vi "IN_1_BIT.vi"(11 "String":string) -> (0 "error out":errorcluster, 3 "data":bool)   [LabVIEW 2017]
uses:
  <vilib>/DAQmx/read.llb/DAQmx Read (Digital Bool 1Line 1Point).vi
  <vilib>/DAQmx/create/channels.llb/DAQmx Create Channel (DO-Digital Output).vi
  <vilib>/DAQmx/miscellaneous.llb/DAQmx Fill In Error Info.vi
panel:
  in  "lines":tag
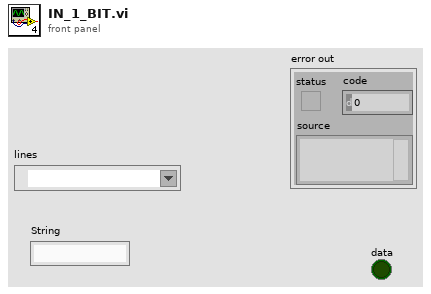
[diagram p1: front panel]
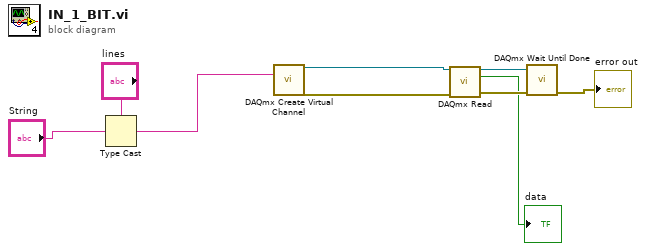
[diagram p0: block diagram]
diagram:
  n1 = Type Cast(type="lines", x="String") -> (*(type *) &x=w7:tag)
  n2 = call-poly <vilib>:"DAQmx Create Virtual Channel.vi"("lines"=w7) -> ("task out"=w5:refnum<k21>, "error out"=w4:errorcluster)  [unwired: 13 in]
  n3 = call-poly <vilib>:"DAQmx Read.vi"("task/channels in"=w5, "error in"=w4) -> ("task out"=w3:refnum<k21>, "data"=→"data":bool, "error out"=w2:errorcluster)  [unwired: 11 in]
  n4 = call <vilib>:"DAQmx Wait Until Done.vi"("task/channels in"=w3, "error in"=w2) -> ("error out"=→"error out":errorcluster)  [unwired: 12 in, 1 out]
